vi "Init Tree.vi"(8 "error in (no error)":errorcluster, 10 "Tree Reference In":refnum<vi>, 11 "CS++MessageMakerMain in":refnum<class "CS++MessageMakerMain.lvclass">) -> (0 "error out":errorcluster, 2 "Tree Reference Out":refnum<vi>, 3 "CS++MessageMakerMain out":refnum<class "CS++MessageMakerMain.lvclass">)   [LabVIEW 2014, in "CS++MessageMakerMain.lvlib" / "CS++MessageMakerMain.lvclass"]
uses:
  CS++MessageMakerMain.lvclass
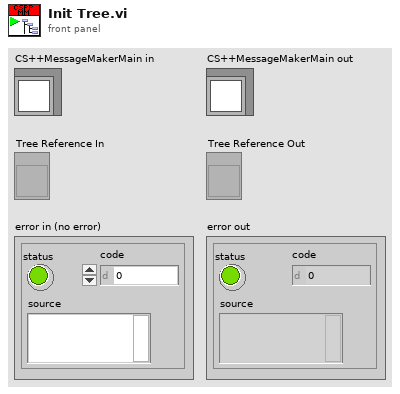
[diagram p1: front panel]
types:
  T1 = typedef "imagedata.ctl" = cluster{"image type":i32, "image depth":i32, "image":u8[], "mask":u8[], "colors":u32[], "Rectangle":cluster{"left":i16, "top":i16, "right":i16, "bottom":i16}}
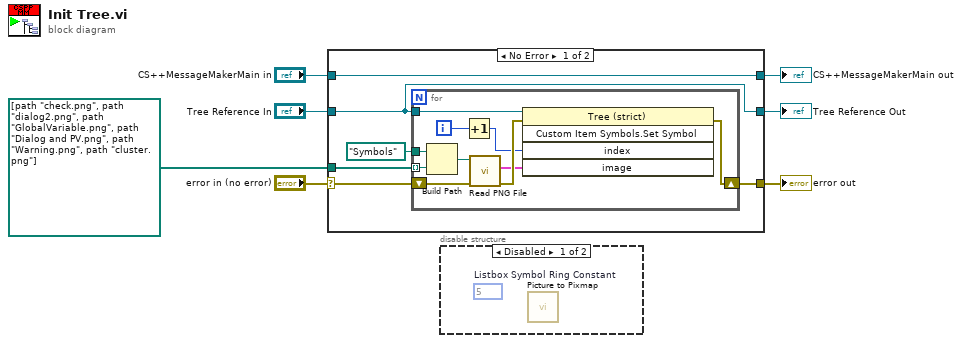
[diagram p0: block diagram]
diagram:
  n1 = case shown="No Error" "error in (no error)" {
    selector: "error in (no error)" -> [w12 w26]
    tunnel: [w11 w26] -> w6
    tunnel: [w13 w25] -> w4
    tunnel: "CS++MessageMakerMain in" -> [w13 w25]
    tunnel: "Tree Reference In" -> [w10 w24]
    tunnel: [w10 w24] -> w2
    tunnel: path[] [path "check.png", path "dialog2.png", path "GlobalVariable.png", path "Dialog and PV.png", path "Warning.png", path "cluster.png"] -> [w9 _]
    frame No Error {
      n2 = for {
        shift-right: [w21] -> w11
        shift-left: w12 -> [w23]
        tunnel: w10 -> [w19]
        tunnel: w9 -> [w15] mode=indexing
        tunnel: path "Symbols" ("Path to PNG file for symbol") -> [w14]
        i -> [w18]
        n3 = Build Path(base path=w14, name or relative path=w15) -> (appended path=w16:path)
        n4 = Increment(x=w18) -> (x+1=w17:i32)
        n5 = call <vilib>:"Read PNG File.vi"("error in (no error)"=w23, "path to PNG file"=w16) -> ("error out"=w22:errorcluster, "image data"=w20:T1)  [unwired: 7 in, 1 out]
        n6 = invoke class="Tree (strict)" method="Custom Item Symbols.Set Symbol"(reference=w19, error in=w22, "index"=w17, "image"=w20) -> (error out=w21:errorcluster)  [unwired: 1 in, 4 out]
      }
    }
    frame Error {
    }
  }
  "error out" <- w6
  "CS++MessageMakerMain out" <- w4
  "Tree Reference Out" <- w2
  n7 = disable-structure shown="Disabled" {
    frame Disabled {
      (unwired) 5  # Listbox Symbol Ring Constant
      n8 = call <vilib>:"Picture to Pixmap.vi"() -> ()  [unwired: 10 in, 2 out]
    }
    frame Enabled {
    }
  }
